vi "BaseProvider_GetStaticMethods.vi"(1 "ClassTemplateName":string, 3 "ConnectorPaneSettings":string, 5 "error in":errorcluster) -> (15 "NormalMethods":T1[](array[typedef]), 19 "error out":errorcluster)   [LabVIEW 2014]
uses:
  <resource>/Framework/Providers/Open_GDS/ClassProviders/Provider_LvNativeClass/ClassWriterNative_class/MethodInfo.ctl
  <resource>/Framework/Providers/Open_GDS/ClassProviders/Provider_LvNativeClass/ClassWriterNative_class/MethodType.ctl
  <vilib>/Utility/config.llb/Read Key (String).vi
  <vilib>/Utility/config.llb/NI_LVConfig.lvlib
  <resource>/Framework/Providers/Open_GDS/ClassProviders/Provider_LvNativeClass/ClassWriterNative_class/ClassWriterNative.lvclass
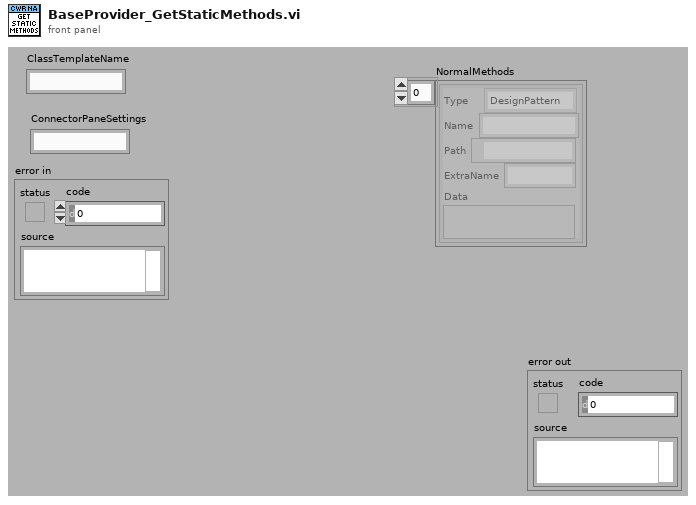
[diagram p1: front panel]
types:
  T1 = typedef "ClassWriterNative.lvclass/MethodInfo.ctl" = cluster{"Type":T2, "Name":string, "Path":path, "ExtraName":string, "Data":variant}
  T2 = typedef "ClassWriterNative.lvclass/MethodType.ctl" = enum16{"Normal", "MethodPlugIn", "DesignPattern", "AF-Method"}
  T3 = typedef "NI_LVConfig.lvlib/Config Data RefNum.ctl" = refnum<k1>
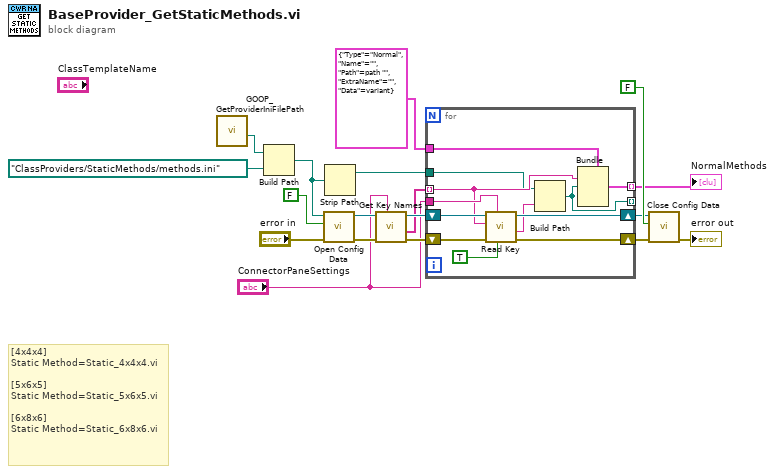
[diagram p0: block diagram]
diagram:
  # "[4x4x4]\nStatic Method=Static_4x4x4.vi\n\n[5x6x5]\nStatic Method=Static_5x6x5.vi\n\n[6x8x6]\nStatic Method=Static_6x8x6.vi"
  n1 = call <resource>:"GOOP_GetProviderIniFilePath.vi"() -> ("ProviderMainFolder"=w15:path)  [unwired: 10 in, 1 out]
  n2 = Build Path(base path=w15, name or relative path=path "ClassProviders/StaticMethods/methods.ini" ("base path")) -> (appended path=w3:path)
  n3 = call <vilib>:"Open Config Data.vi"("error in (no error)"="error in", "create file if necessary (T)"=FALSE ("create file if necessary? (T)"), "configuration file path"=w3) -> ("error out"=w9:errorcluster, "refnum"=w8:T3)  [unwired: 6 in, 1 out]
  n4 = Strip Path(path=w3) -> (stripped path=w2:path)  [unwired: 1 out]
  n5 = call <vilib>:"Get Key Names.vi"("section"="ConnectorPaneSettings", "error in (no error)"=w9, "refnum"=w8) -> ("error out"=w7:errorcluster, "key names"=w5:string[], "refnum out"=w6:T3)  [unwired: 5 in, 1 out]
  n6 = for {
    shift-right: [w26] -> w11
    shift-left: w7 -> [w29]
    shift-right: [w27] -> w12
    shift-left: w6 -> [w30]
    tunnel: "ConnectorPaneSettings" -> [w28]
    tunnel: w5 -> [w22] mode=indexing
    tunnel: [w24] -> w1 mode=indexing
    tunnel: T1 {"Type"=enum."Normal", "Name"="", "Path"=path "", "ExtraName"="", "Data"=variant} ("Cluster") -> [w25]
    tunnel: [w19] -> _ mode=indexing
    tunnel: w2 -> [w21]
    n7 = call-poly <vilib>:"Read Key.vi"("read raw string? (F)"=TRUE, "section"=w28, "error in (no error)"=w29, "key"=w22, "refnum"=w30) -> ("error out"=w26:errorcluster, "value"=w20:string, "refnum out"=w27:T3)  [unwired: 3 in, 1 out]
    n8 = Build Path(base path=w21, name or relative path=w20) -> (appended path=w19:path)
    n9 = Bundle(cluster=w25, "Name"=w22, "Path"=w19) -> (w24:T1)  [unwired: 3 in]
  }
  "NormalMethods" <- w1
  n10 = call <vilib>:"Close Config Data.vi"("error in (no error)"=w11, "write file if changed (T)"=FALSE ("create file if necessary? (T)"), "refnum"=w12) -> ("error out"=→"error out":errorcluster)  [unwired: 7 in, 1 out]
